vi "LightFieldBackgroundNaming.vi"(8 "Cycle time\n(ms)":i32=3 min=0 step=1, 9 "On CCD Acc.":i32=3 min=0 step=1, 10 "BIN":u16(ring)=2 items=["1x1", "2x2", "4x4"], 11 "MODE":u16(ring) items=["Normal", "DIF"]) -> (1 "FilePath":string, 2 "Exists":bool, 3 "Background File Name":string)   [LabVIEW 2018]
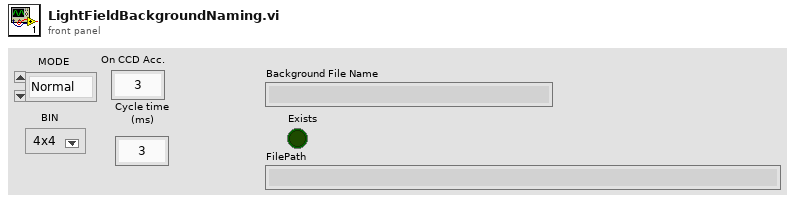
[diagram p1: front panel]
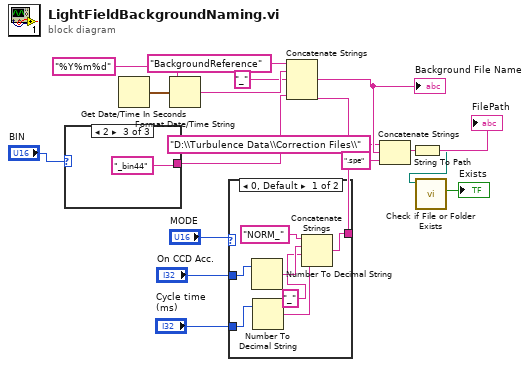
[diagram p0: block diagram]
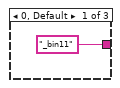
[diagram p2: hidden frame]
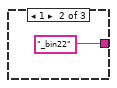
[diagram p3: hidden frame]
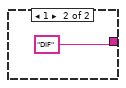
[diagram p4: hidden frame]
diagram:
  n1 = case shown="2" "BIN" {
    tunnel: ["_bin11" "_bin22" "_bin44"] -> w8
    frame 0, Default {
    }
    frame 1 {
    }
    frame 2 {
    }
  }
  n2 = Get Date/Time In Seconds() -> (seconds since 1Jan1904=w16:timestamp)
  n3 = Format Date/Time String(time format string (%c)="%Y%m%d", seconds (now)=w16) -> (date/time string=w14:string)  [unwired: 1 in]
  n4 = case shown="0, Default" "MODE" {
    tunnel: [w26 "DIF"] -> w12
    tunnel: "On CCD Acc." -> [w25 _]
    tunnel: "Cycle time\n(ms)" -> [w23 _]
    frame 0, Default {
      n5 = Number To Decimal String(number=w25) -> (decimal integer string=w24:string)  [unwired: 1 in]
      n6 = Number To Decimal String(number=w23) -> (decimal integer string=w22:string)  [unwired: 1 in]
      n7 = Concatenate Strings("NORM_", w24, "_" ("string"), w22) -> (w26:string)
    }
    frame 1 {
    }
  }
  n8 = Concatenate Strings("BackgroundReference" ("string"), w14, "_" ("string"), w12, w8) -> (w4:string)
  "Background File Name" <- w4
  n9 = Concatenate Strings("D:\\Turbulence Data\\Correction Files\\" ("string"), w4, ".spe" ("string")) -> (w7:string)
  "FilePath" <- w7
  n10 = String To Path(string=w7) -> (path=w6:path)
  n11 = call "Check if File or Folder Exists.vi"("path"=w6) -> ("file or folder exists?"=→"Exists":bool)  [unwired: 8 in, 2 out]
